vi "ZE_Recorder_ReadFromTasks.vi"(8 "error in":errorcluster, 9 "sampling rate":dbl=-1.0, 10 "No of channels":i16, 11 "ACK Tasks":refnum<k21>[](array[refnum])) -> (0 "error out":errorcluster, 3 "data":dbl[][](array[numeric]))   [LabVIEW 2025, in "ZE_Recorder.lvlib"]
doc: "ZE_Recorder_ReadFromTasks.vi\n----------------------------------------------\nThe VI reads the data from the task array as either 1D or 2D data.\n\nInputs:\n---------------------\n- error in : Cluster; \n- sampling rate : DBL; \n- No of channels : I16; \n- ACK Tasks : 1DArrayOfRefnum; \n\nOutputs:\n---------------------\n- error out : Cluster; \n- data : 2DArrayOfDBL; \n\n----------------------------------------------\n25.12.2017\nZühlke Engineering AG\nCH-8952 Schlieren\nwww.zuehlke.com"
uses:
  ZE_Recorder.lvlib
  <vilib>/DAQmx/read.llb/DAQmx Read (Analog 1D DBL 1Chan NSamp).vi
  <vilib>/DAQmx/read.llb/DAQmx Read (Analog 2D DBL NChan NSamp).vi
  <vilib>/DAQmx/miscellaneous.llb/DAQmx Fill In Error Info.vi
  <resource>/objmgr/daqmx.rc
panel:
  # "Connector Pane"
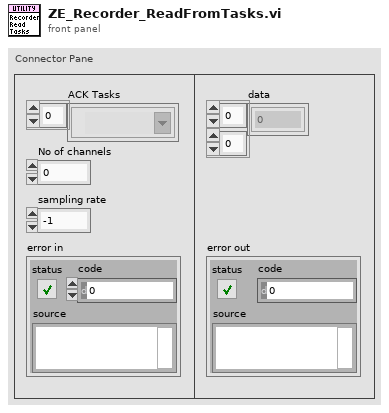
[diagram p1: front panel]
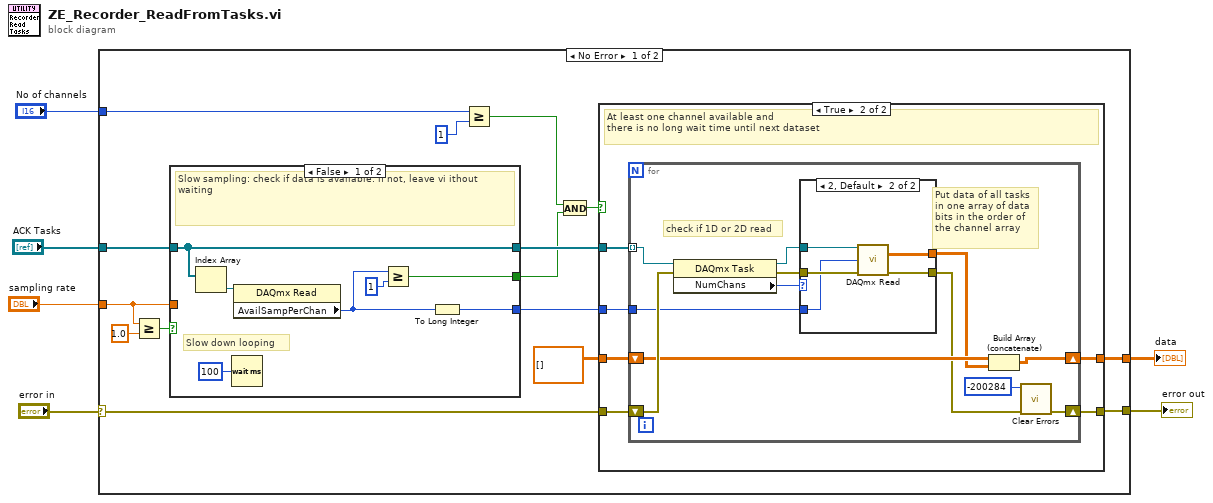
[diagram p0: block diagram]
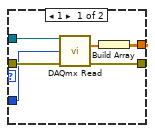
[diagram p3: hidden frame]
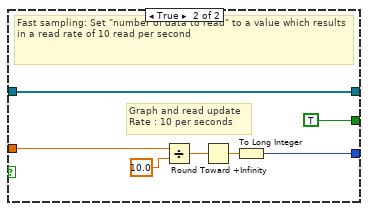
[diagram p4: hidden frame]
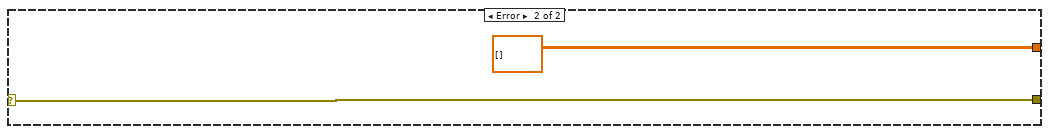
[diagram p5: hidden frame]
diagram:
  n1 = case shown="No Error" "error in" {
    selector: "error in" -> [w17 w68]
    tunnel: [w21 dbl[][] []] -> w6
    tunnel: [w16 w68] -> w5
    tunnel: "No of channels" -> [w20 _]
    tunnel: "ACK Tasks" -> [w10 _]
    tunnel: "sampling rate" -> [w13 _]
    frame No Error {
      n2 = Greater Or Equal?(x=w13, y=1.0) -> (x >= y?=w12:bool)
      n3 = case shown="False" w12 {
        tunnel: [w53 w63] -> w14
        tunnel: w13 -> [_ w62]
        tunnel: [w59 w61] -> w9
        tunnel: w10 -> [w59 w61]
        tunnel: [w55 TRUE] -> w7
        frame False {
          # "Slow down looping"
          # "Slow sampling: check if data is available. if not, leave vi ithout waiting"
          n4 = Index Array(array=w59) -> (element=w58:refnum<k21>)  [unwired: 1 in]
          n5 = Wait (ms)(milliseconds to wait=u32 100) -> ()  [unwired: 1 out]
          n6 = property class="DAQmx Read"(reference=w58) -> ("AvailSampPerChan"=w54:u32)  [unwired: 1 in, 2 out]
          n7 = Greater Or Equal?(x=w54, y=u32 1) -> (x >= y?=w55:bool)
          n8 = To Long Integer(number=w54) -> (32bit integer=w53:i32)
        }
        frame True {
          # "Graph and read update\nRate : 10 per seconds"
          # "Fast sampling: Set \"number of data to read\" to a value which results in a read rate of 10 read per second"
          n9 = Divide(x=w62, y=10.0) -> (x/y=w65:dbl)
          n10 = Round Toward +Infinity(x=w65) -> (ceil(x): smallest int >= x=w64:dbl)
          n11 = To Long Integer(number=w64) -> (32bit integer=w63:i32)
        }
      }
      n12 = Greater Or Equal?(x=w20, y=i16 1 ("No of channels")) -> (x >= y?=w18:bool)
      n13 = And(x=w18, y=w7) -> (x .and. y?=w8:bool)
      n14 = case shown="True" w8 {
        tunnel: [w22 w29] -> w21
        tunnel: w9 -> [_ w28]
        tunnel: w17 -> [w23 w27]
        tunnel: [w23 w26] -> w16
        tunnel: dbl[][] [] ("data") -> [w22 w25]
        tunnel: w14 -> [_ w24]
        frame False {
        }
        frame True {
          # "At least one channel available and\nthere is no long wait time until next dataset"
          n15 = for {
            shift-right: [w31] -> w26
            shift-left: w27 -> [w39]
            tunnel: w28 -> [w41] mode=indexing
            shift-right: [w34] -> w29
            shift-left: w25 -> [w36]
            tunnel: w24 -> [w33]
            # "Put data of all tasks\nin one array of data\nbits in the order of\nthe channel array"
            # "check if 1D or 2D read"
            n16 = property class="DAQmx Task"(reference=w41, error in=w39) -> (reference out=w37:refnum<k21>, error out=w38:errorcluster, "NumChans"=w40:u32)
            n17 = case shown="2, Default" w40 {
              tunnel: w37 -> [w47 w52]
              tunnel: [w44 w50] -> w35
              tunnel: [w45 w51] -> w32
              tunnel: w38 -> [w43 w49]
              tunnel: w33 -> [w42 w48]
              frame 1 {
                n18 = call-poly <vilib>:"DAQmx Read.vi"("task/channels in"=w47, "number of samples per channel"=w42, "error in"=w43) -> ("data"=w46:dbl[], "error out"=w45:errorcluster)  [unwired: 10 in, 1 out]
                n19 = Build Array(w46) -> (w44:dbl[][])
              }
              frame 2, Default {
                n20 = call-poly <vilib>:"DAQmx Read.vi"("task/channels in"=w52, "number of samples per channel"=w48, "error in"=w49) -> ("data"=w50:dbl[][], "error out"=w51:errorcluster)  [unwired: 10 in, 1 out]
              }
            }
            n21 = Build Array (concatenate)(w36, w35) -> (w34:dbl[][])
            n22 = call <vilib>:"Clear Errors.vi"("error in (no error)"=w32, "specific error code to clear (0: all)"=-200284) -> ("error out"=w31:errorcluster)  [unwired: 4 in, 1 out]
          }
        }
      }
    }
    frame Error {
    }
  }
  "data" <- w6
  "error out" <- w5
